vi "DataLoggerCSV.vi"(6 "Queue In":refnum<queue>, 7 "Error In":errorcluster, 8 "String Path In":string, 9 "Log State In":T1, 10 "File Ref In":refnum<file>) -> (0 "Error Out":errorcluster, 1 "String Path Out":string, 2 "Log State Out":T1, 3 "File Ref Out":refnum<file>)   [LabVIEW 2013]
uses:
  eng/trunk/ni/cRIO Master Files/Controls/LogState.ctl
  <vilib>/Utility/file.llb/Write To Spreadsheet File (DBL).vi
  <vilib>/Utility/file.llb/Write To Spreadsheet File (string).vi
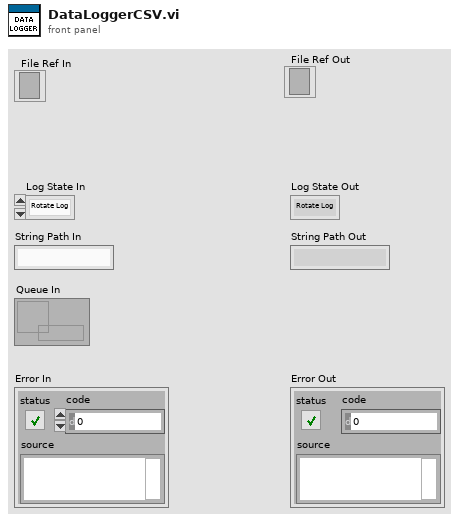
[diagram p1: front panel]
types:
  T1 = typedef "LogState.ctl" = enum16{"Rotate Log", "Log Data", "Wait", "Close File", "Generate Filename", "Create New File"}
  T2 = enum16{"open", "replace", "create", "open or create", "replace or create", "replace or create with confirmation"}
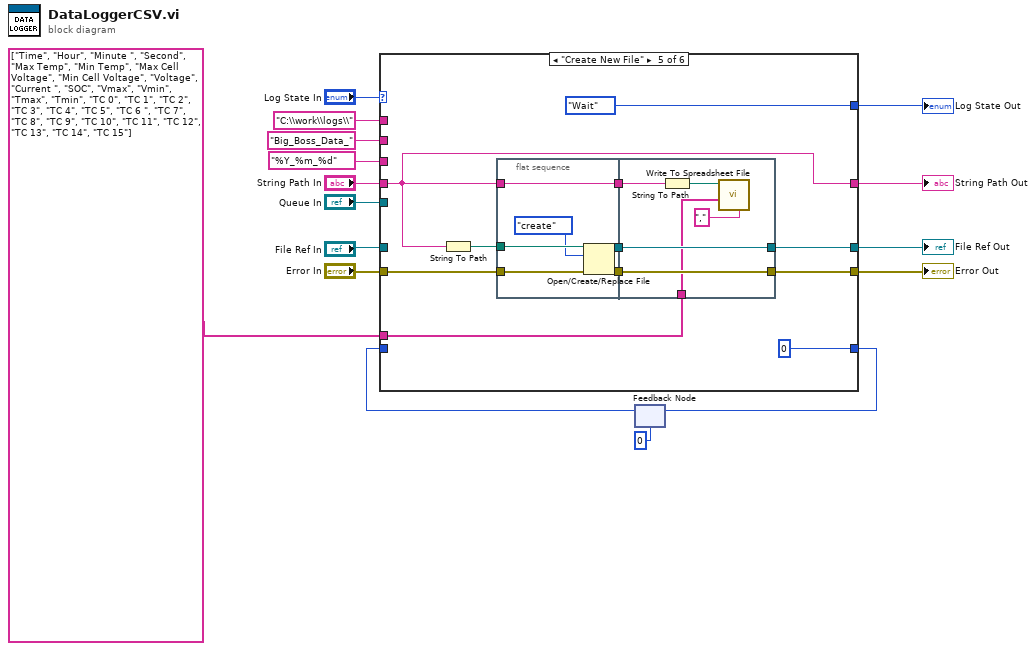
[diagram p0: block diagram]
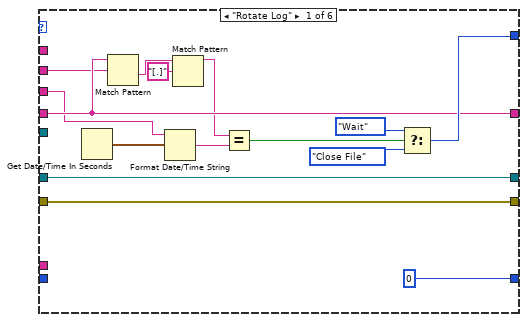
[diagram p2: hidden frame]
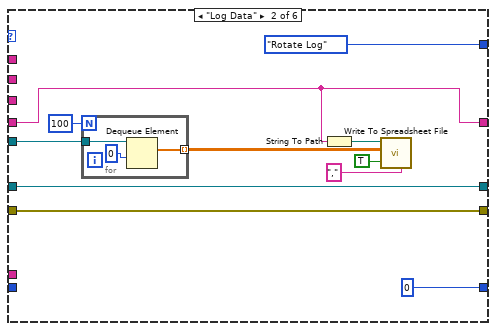
[diagram p3: hidden frame]
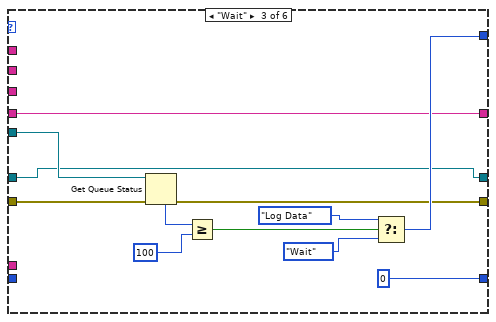
[diagram p4: hidden frame]
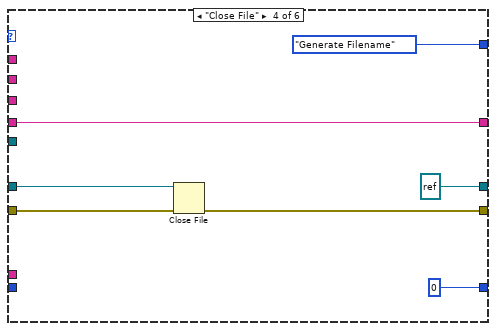
[diagram p5: hidden frame]
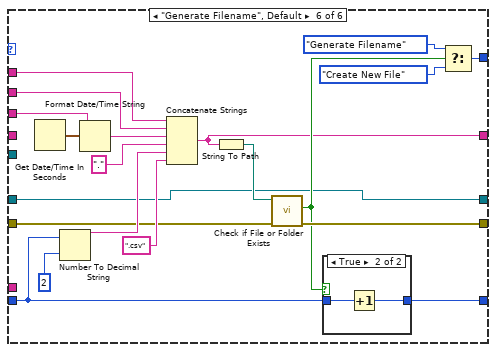
[diagram p6: hidden frame]
diagram:
  n1 = feedback #1(0 ("Filename Counter")) -> (w3:i32)
  n2 = case shown="\"Create New File\"" "Log State In" {
    tunnel: "Error In" -> [w27 w34 w55 w61 w74 w98]
    tunnel: [w27 w34 w49 w60 w71 w97] -> w11
    tunnel: "Queue In" -> [_ w41 w54 _ _ _]
    tunnel: [w31 LogState."Rotate Log" ("Log State") w53 LogState."Generate Filename" ("Log State") LogState."Wait" ("Log State") w100] -> w10
    tunnel: [w26 w37 w48 w58 w65 w92] -> w12
    tunnel: "String Path In" -> [w26 w37 w48 w58 w65 _]
    tunnel: w3 -> [_ _ _ _ _ w95]
    tunnel: [0 ("Filename Counter") 0 ("Filename Counter") 0 ("Filename Counter") 0 ("Filename Counter") 0 ("Filename Counter") w93] -> w4
    tunnel: "C:\\work\\logs\\" ("string") -> [_ _ _ _ _ w90]
    tunnel: "%Y_%m_%d" ("time format string (%c)") -> [w21 _ _ _ _ w91]
    tunnel: "Big_Boss_Data_" ("string") -> [w18 _ _ _ _ w89]
    tunnel: [w17 w33 w46 refnum<file> refnum ("File Ref In") w70 w88] -> w6
    tunnel: "File Ref In" -> [w17 w33 w46 w62 _ w88]
    tunnel: string[] ["Time", "Hour", "Minute ", "Second", "Max Temp", "Min Temp", "Max Cell Voltage", "Min Cell Voltage", "Voltage", "Current ", "SOC", "Vmax", "Vmin", "Tmax", "Tmin", "TC 0", "TC 1", "TC 2", "TC 3", "TC 4", "TC 5", "TC 6 ", "TC 7", "TC 8", "TC 9", "TC 10", "TC 11", "TC 12", "TC 13", "TC 14", "TC 15"] ("channel name(s) in (Untitled)") -> [_ _ _ _ w67 _]
    frame "Rotate Log" {
      n3 = Get Date/Time In Seconds() -> (seconds since 1Jan1904=w23:timestamp)
      n4 = Match Pattern(string=w26, regular expression=w18) -> (after substring=w25:string)  [unwired: 1 in, 3 out]
      n5 = Format Date/Time String(time format string (%c)=w21, seconds (now)=w23) -> (date/time string=w20:string)  [unwired: 1 in]
      n6 = Match Pattern(string=w25, regular expression="[.]") -> (before substring=w19:string)  [unwired: 1 in, 3 out]
      n7 = Equal?(x=w19, y=w20) -> (x = y?=w22:bool)
      n8 = Select(t=LogState."Wait" ("Log State"), s=w22, f=LogState."Close File" ("Log State")) -> (s? t:f=w31:T1)
    }
    frame "Log Data" {
      n9 = for {
        N: 100 -> [_]
        tunnel: w41 -> [w44]
        tunnel: [w43] -> w36 mode=indexing
        n10 = Dequeue Element(queue=w44, timeout in ms (-1)=0) -> (element=w43:dbl[])  [unwired: 1 in, 3 out]
      }
      n11 = String To Path(string=w37) -> (path=w38:path)
      n12 = call-poly <vilib>:"Write To Spreadsheet File.vi"("delimiter (\\t)"="," ("delimiter (\\t)"), "append to file? (new file:F)"=TRUE, "2D data"=w36, "file path (dialog if empty)"=w38) -> ()  [unwired: 4 in, 1 out]
    }
    frame "Wait" {
      n13 = Get Queue Status(queue=w54, error in (no error)=w55) -> (error out=w49:errorcluster, # elements in queue=w57:i32)  [unwired: 1 in, 6 out]
      n14 = Greater Or Equal?(x=w57, y=100) -> (x >= y?=w50:bool)
      n15 = Select(t=LogState."Log Data" ("Log State"), s=w50, f=LogState."Wait" ("Log State")) -> (s? t:f=w53:T1)
    }
    frame "Close File" {
      n16 = Close File(refnum=w62, error in=w61) -> (error out=w60:errorcluster)  [unwired: 1 out]
    }
    frame "Create New File" {
      n17 = String To Path(string=w65) -> (path=w73:path)
      n18 = flat-sequence {
        tunnel: w74 -> [w81]
        tunnel: w73 -> [w80]
        tunnel: [w79] -> w69
        tunnel: [w78] -> w68
        tunnel: w65 -> [w76]
        tunnel: [w76] -> w66
        tunnel: [w86] -> w70
        tunnel: [w87] -> w71
        tunnel: w69 -> [w87]
        tunnel: w68 -> [w86]
        tunnel: w67 -> [w83]
        tunnel: w66 -> [w82]
        frame #0 {
          n19 = Open/Create/Replace File(file path (use dialog)=w80, error in=w81, operation (0:open)=T2."create") -> (refnum out=w78:refnum<file>, error out=w79:errorcluster)  [unwired: 3 in, 1 out]
        }
        frame #1 {
          n20 = String To Path(string=w82) -> (path=w84:path)
          n21 = call-poly <vilib>:"Write To Spreadsheet File.vi"("delimiter (\\t)"="," ("delimiter (\\t)"), "1D data"=w83, "file path (dialog if empty)"=w84) -> ()  [unwired: 5 in, 1 out]
        }
      }
    }
    frame "Generate Filename", Default {
      n22 = Get Date/Time In Seconds() -> (seconds since 1Jan1904=w107:timestamp)
      n23 = Number To Decimal String(number=w95, width (-)=i16 2) -> (decimal integer string=w101:string)
      n24 = Format Date/Time String(time format string (%c)=w91, seconds (now)=w107) -> (date/time string=w106:string)  [unwired: 1 in]
      n25 = Concatenate Strings(w90, w89, w106, "." ("string"), w101, ".csv" ("string")) -> (w92:string)
      n26 = String To Path(string=w92) -> (path=w105:path)
      n27 = call <vilib>:"Check if File or Folder Exists.vi"("error in (no error)"=w98, "path"=w105) -> ("error out"=w97:errorcluster, "file or folder exists?"=w94:bool)  [unwired: 7 in, 1 out]
      n28 = case shown="True" w94 {
        tunnel: w95 -> [w108 w109]
        tunnel: [w108 w110] -> w93
        frame False {
        }
        frame True {
          n29 = Increment(x=w109) -> (x+1=w110:i32)
        }
      }
      n30 = Select(t=LogState."Generate Filename" ("Log State Out"), s=w94, f=LogState."Create New File" ("Log State Out")) -> (s? t:f=w100:T1)
    }
  }
  "String Path Out" <- w12
  "Error Out" <- w11
  "Log State Out" <- w10
  "File Ref Out" <- w6
  n31 = feedback-in #1(w4) -> ()
